vi "DeCompress.vi"(8 "错误输入":errorcluster, 11 "Compressed String":string) -> (0 "错误输出":errorcluster, 3 "DeCompressed String":string)   [LabVIEW 2012, in "GZip.lvlib"]
uses:
  GZip.lvlib
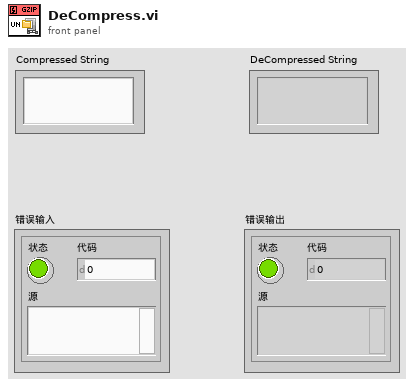
[diagram p1: front panel]
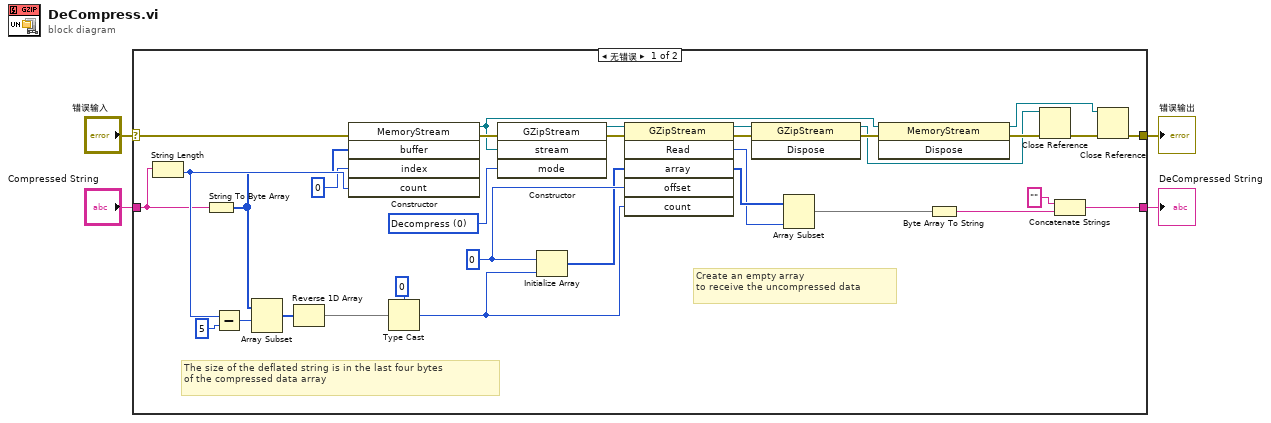
[diagram p0: block diagram]
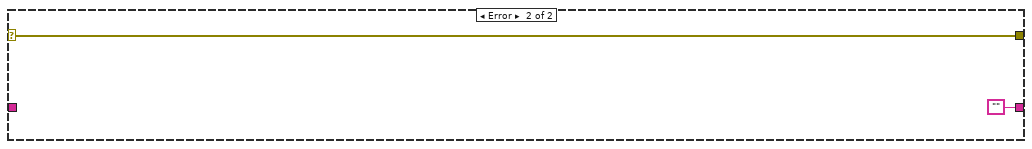
[diagram p2: hidden frame]
diagram:
  n1 = case shown="无错误" "错误输入" {
    selector: "错误输入" -> [w7 w38]
    tunnel: "Compressed String" -> [w5 _]
    tunnel: [w28 ""] -> w1
    tunnel: [w11 w38] -> w2
    frame No Error {
      w17 = u8 0 ("offset")
      w20 = 0 items=["Decompress", "Compress"] ("mode")
      # "Create an empty array \nto receive the uncompressed data"
      # "The size of the deflated string is in the last four bytes \nof the compressed data array"
      n2 = String Length(string=w5) -> (length=w29:i32)
      n3 = String To Byte Array(string=w5) -> (unsigned byte array=w6:u8[])
      n4 = Subtract(x=w29, y=5) -> (x-y=w31:i32)
      n5 = Array Subset(array=w6, index=w31) -> (w32:u8[])  [unwired: 1 in]
      n6 = Reverse 1D Array(array=w32) -> (reversed array=w33:u8[])
      n7 = constructor class="MemoryStream"(error in=w7, "buffer"=w6, "index"=0, "count"=w29) -> (reference out=w19:refnum<k24>, error out=w36:errorcluster)  [unwired: 2 in, 4 out]
      n8 = Type Cast(type=u32 0, x=w33) -> (*(type *) &x=w35:u32)
      n9 = constructor class="GZipStream"(error in=w36, "stream"=w19, "mode"=w20) -> (reference out=w22:refnum<k24>, error out=w23:errorcluster)  [unwired: 2 in, 3 out]
      n10 = Initialize Array(w17, w35) -> (w16:u8[])
      n11 = invoke class="GZipStream" method="Read"(reference=w22, error in=w23, "array"=w16, "offset"=w17, "count"=w35) -> (reference out=w21:refnum<k24>, error out=w24:errorcluster, "Read"=w13:i32, "array"=w18:u8[])  [unwired: 1 in, 2 out]
      n12 = invoke class="GZipStream" method="Dispose"(reference=w21, error in=w24) -> (reference out=w8:refnum<k24>, error out=w25:errorcluster)  [unwired: 1 in, 1 out]
      n13 = Array Subset(array=w18, length=w13) -> (w14:u8[])  [unwired: 1 in]
      n14 = invoke class="MemoryStream" method="Dispose"(reference=w19, error in=w25) -> (reference out=w12:refnum<k24>, error out=w10:errorcluster)  [unwired: 1 in, 1 out]
      n15 = Byte Array To String(unsigned byte array=w14) -> (string=w15:string)
      n16 = Close Reference(reference=w8, error in (no error)=w10) -> (error out=w9:errorcluster)
      n17 = Concatenate Strings("", w15) -> (w28:string)
      n18 = Close Reference(reference=w12, error in (no error)=w9) -> (error out=w11:errorcluster)
    }
    frame Error {
    }
  }
  "错误输出" <- w2
  "DeCompressed String" <- w1
